vi "Metronome.vi"() -> ()   [LabVIEW 2014]
panel:
  in  "Stop":bool
  in  "Beats Per Minute":dbl
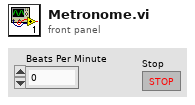
[diagram p1: front panel]
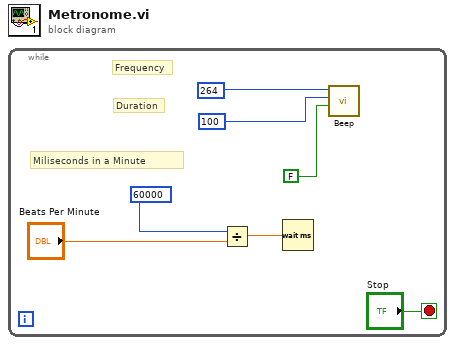
[diagram p0: block diagram]
diagram:
  n1 = while {
    stop <- "Stop" stop-if-true
    # "Duration"
    # "Frequency"
    # "Miliseconds in a Minute"
    n2 = Divide(x=60000, y="Beats Per Minute") -> (x/y=w4:dbl)
    n3 = Wait (ms)(milliseconds to wait=w4) -> ()  [unwired: 1 out]
    n4 = call <vilib>:"Beep.vi"("use system alert? (T) - ignored"=FALSE ("use system alert? (T)"), "duration (msec) - ignored"=u32 100 ("duration (msec)"), "frequency (Hz) - ignored"=u32 264 ("frequency (Hz)")) -> ()  [unwired: 9 in]
  }
